vi "str to strarray.vi"(2 "String":string) -> (6 "str array":string[](array[string]))   [LabVIEW 2013, in "CreateOPCUAServerAuto.lvlib"]
uses:
  CreateOPCUAServerAuto.lvlib
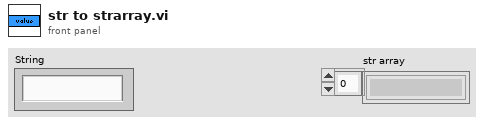
[diagram p1: front panel]
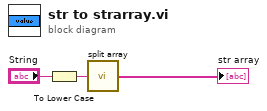
[diagram p0: block diagram]
diagram:
  n1 = To Lower Case(string="String") -> (all lower case string=w2:string)
  n2 = call "split array.vi"("string"=w2) -> ("split arr"=→"str array":string[])  [unwired: 8 in]
